vi "nameArray.vi"(8 "error in":errorcluster) -> (0 "error out":errorcluster, 2 "Array":T1[][](array[typedef]))   [LabVIEW 2020]
uses:
  _controls/element.ctl
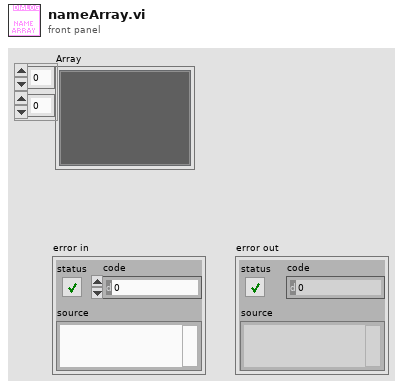
[diagram p1: front panel]
types:
  T1 = typedef "element.ctl" = cluster{"Color Box":u32, "label":string}
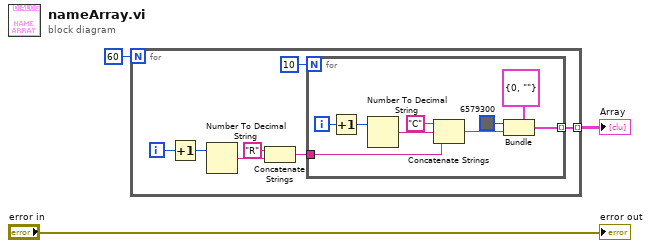
[diagram p0: block diagram]
diagram:
  n1 = for {
    N: 60 -> [_]
    tunnel: [w7] -> w3 mode=indexing
    i -> [w9]
    n2 = Increment(x=w9) -> (x+1=w6:i32)
    n3 = Number To Decimal String(number=w6) -> (decimal integer string=w8:string)  [unwired: 1 in]
    n4 = Concatenate Strings("R" ("string"), w8) -> (w5:string)
    n5 = for {
      N: 10 -> [_]
      tunnel: w5 -> [w15]
      tunnel: [w16] -> w7 mode=indexing
      i -> [w12]
      n6 = Increment(x=w12) -> (x+1=w13:i32)
      n7 = Number To Decimal String(number=w13) -> (decimal integer string=w11:string)  [unwired: 1 in]
      n8 = Concatenate Strings("C" ("string"), w11, w15) -> (w19:string)
      n9 = Bundle(cluster=T1 {"Color Box"=0, "label"=""} ("element"), "Color Box"=u32 6579300, "label"=w19) -> (w16:T1)
    }
  }
  "Array" <- w3
  "error out" <- "error in"
